vi "PAM v1.2.vi"() -> ()   [LabVIEW 2011]
uses:
  PAM_Control.ctl
  <vilib>/Utility/error.llb/DialogType.ctl
  <vilib>/Analysis/Matrix/Datatypes/RealMatrix.ctl
  <vilib>/DAQmx/read.llb/DAQmx Read (Analog 1D Wfm NChan NSamp).vi
  <vilib>/DAQmx/write.llb/DAQmx Write (Analog 1D DBL NChan 1Samp).vi
  PAM SubVIs/RH Probe Global Var.vi
  <vilib>/DAQmx/configure/timing.llb/DAQmx Timing (Sample Clock).vi
  <vilib>/Utility/file.llb/Write To Spreadsheet File (string).vi
  <vilib>/Analysis/Matrix/Numeric/Conversions/Matrix To Array - RM.vi
  <vilib>/DAQmx/miscellaneous.llb/DAQmx Fill In Error Info.vi
  Program Files (x86)/National Instruments/LabVIEW 2011/resource/objmgr/daqmx.rc
  <vilib>/Analysis/Matrix/NI_Matrix.lvlib
panel:
  out "O3 Data":sgl[](graph)
  out "SO2 Data":sgl[](graph)
  out "NO, NO2, NOx Data":dbl[][](graph)
  out "Bad Advantech Data Points":dbl
  out "Run In Progress?":bool
  out "Manual":bool
  in  "MFC Sequence File":path=path "C:/Users/PAM/Dropbox/Research - Dr. Williams/PAM/LabVIEW PAM/PAM Edited/defaultMFCSequence.txt"
  out "Auto":bool
  out "P Unit":string
  out "Pressure Transducer":dbl(knob) scale=1.9345053227622008e-18..193.3373735517042
  out "Error Out":errorcluster
  out "Elapsed Time (min)":dbl format="%#_2g"
  in  "Run Start Time":timestamp format="%<%X\n%x>T"
  out "NOx Units":string="LPM"
  in  "NOx Control (LPM)":dbl(slide) scale=0.0..0.04
  out "NOx Reading (LPM) 3":dbl(slide) scale=0.0..0.5
  out "VOC Units":string="LPM"
  in  "VOC Control (LPM)":dbl(slide) scale=0.0..0.5
  out "VOC Reading (LPM)":dbl(slide) scale=0.0..0.04
  out "O2 Units":string="LPM"
  in  "O2 Control (LPM)":dbl(slide) scale=0.0..1.0
  out "O2 Reading (LPM) 2":dbl(slide) scale=0.0..1.0 scale format="%#.2f"
  out "N2 Units":string="LPM"
  in  "N2 Control (LPM)":dbl(slide) scale=0.0..20.0
  out "N2 Reading (LPM)":dbl(slide) scale=0.0..20.0 scale format="%#.2f"
  out "AI (non TC) Units":string[](array[string])
  out "AI (non TC) Names":string[](array[string])
  out "RH Values":dbl[](array[numeric]) format="%#.2f"
  out "All Temp Units":i32[](array[ring]) items=["Deg C"=10143, "Deg F"=10144, "Kelvins"=10325, "Deg R"=10145, "From Custom Scale"=10065]
  out "All TC Labels":string[](array[string])
  out "TC Values Readings":dbl[](array[numeric]) format="%#_3g"
  out "Relative Humidity Data":waveform(dbl)[](graph) caption="Waveform Chart"
  in  "Stop Button":bool
  out "Temperature Data":dynamicdata(graph) caption="Waveform Chart"
  in  "Sampling Frequency (Hz)":dbl=5.0 caption="Delay Time (s)"
  in  "Trigger Type":T1(tab)
  in  "In Use? 11":bool=TRUE
  in  "In Use? 10":bool=TRUE
  in  "In Use? 9":bool=TRUE
  in  "In Use? 8":bool=TRUE
  in  "In Use? 7":bool=TRUE
  in  "In Use? 6":bool=TRUE
  in  "In Use? 5":bool=TRUE
  in  "Adv. TC 7":string="TC 7"
  in  "Adv. TC 6":string="TC 6"
  in  "Adv. TC 5":string="TC 5"
  in  "Adv. TC 4":string="TC 4"
  in  "Adv. TC 3":string="TC 3"
  in  "Adv. TC 2":string="TC 2"
  in  "Adv. TC 1":string="TC 1"
  in  "units":i32(ring)=10143 items=["Deg C"=10143, "Deg F"=10144, "Kelvins"=10325, "Deg R"=10145, "From Custom Scale"=10065]
  in  "In Use? 14":bool=TRUE
  in  "Physical Channel 14":tag="Dev1/ai7"
  in  "TC 14":string="PAM Downstream"
  in  "In Use? 13":bool=TRUE
  in  "Physical Channel 13":tag="Dev1/ai3"
  in  "TC 13":string="Humidifier"
  in  "In Use? 12":bool
  in  "Physical Channel 12":tag="Dev1/ai23"
  in  "TC 12":string="TC 12"
  in  "In Use? 15":bool
  in  "In Use? 14":bool
  in  "In Use? 13":bool
  in  "In Use? 12":bool
  in  "Physical Channel 4":tag="Dev1/ai21"
  in  "TC 4":string="TC 11"
  in  "Physical Channel 3":tag="Dev1/ai17"
  in  "TC 3":string="TC 10"
  in  "Physical Channel 2":tag="Dev1/ai20"
  in  "TC 2":string="TC 9"
  in  "Physical Channel":tag="Dev1/ai16"
  in  "TC 1":string="TC 8"
  in  "Thermocouple Type 1":T2=10073 items=["J"=10072, "K"=10073, "N"=10077, "R"=10082, "S"=10085, "T"=10086, "B"=10047, "E"=10055]
  in  "Min Value (deg C)":dbl
  in  "Max Value (deg C)":dbl=100.0
  in  "CJC Source":i32(ring)=10116 items=["Built-In"=10200, "Constant Value"=10116, "Channel"=10113]
  in  "CJC Value":dbl=25.0 format="%0.2f"
  in  "CJC Channel":refnum<k21>
  in  "In Use? 3":bool=TRUE
  in  "In Use? 4":bool=TRUE
  in  "RHT  2":tag="Dev1/ai5"
  in  "RHT Probe 2":string="RH 2"
  in  "RHT  1":tag="Dev1/ai4"
  in  "RHT Probe 1":string="RH 1"
  in  "In Use? 1":bool=TRUE
  in  "RHT  4":tag="Dev1/ai1"
  in  "RHT Probe 4":string="RHT T2"
  in  "RHT  3":tag="Dev1/ai0"
  in  "RHT Probe 3":string="RHT T1"
  in  "In Use? 2":bool=TRUE
  in  "Vaisala RH Scale":tag="RH Vaisala"
  in  "Vaisala T Scale":tag="RHT - Temp"
  in  "physical channels 4":tag="Dev1/ao3"
  out "Scale for VOC MFC 2":tag="NOx uMFC B"
  out "VOC MFC 2":string="VOC"
  in  "physical channels 3":tag="Dev1/ao2"
  out "Scale for NOx MFC 2":tag="NOx uMFC A"
  out "NOx MFC 2":string="NOx"
  in  "physical channels 2":tag="Dev1/ao1"
  out "Scale for O2 MFC 2":tag="O2 MFC B"
  out "O2 MFC 2":string="O2"
  in  "Scale for VOC MFC":tag="NOx uMFC B"
  in  "VOC MFC Channel":tag="Dev1/ai22"
  in  "VOC MFC":string="VOC"
  in  "Scale for NOx MFC":tag="NOx uMFC A"
  in  "NOx MFC Channel":tag="Dev1/ai18"
  in  "NOx MFC":string="NOx"
  in  "Scale for O2 MFC":tag="O2 MFC B"
  in  "O2 MFC Channel":tag="Dev1/ai6"
  in  "O2 MFC":string="O2"
  in  "Scale for N2 MFC":tag="N2 MFC A"
  in  "N2 MFC Channel":tag="Dev1/ai2"
  in  "N2 MFC":string="N2"
  out "Scale for N2 MFC 2":tag="N2 MFC A"
  out "N2 MFC 2":string="N2"
  in  "physical channels":tag="Dev1/ao0"
  in  "Units":enum16{"Torr", "Psia", "Bar", "kPa"}(ring)=enum."Psia"
  in  "In Use? 16":bool=TRUE
  in  "Pressure Transducer Channel":tag="Dev1/ai19"
  in  "Pressure Transducer Label":string="Pressure"
  in  "In Use? 18":bool=TRUE
  in  "Instrument 3":T3(ring)=enum."O3 (49i)"
  in  "In Use? 17":bool=TRUE
  in  "Instrument 2":T3(ring)=enum."SO2 (43i-TLE)"
  in  "In Use? 17":bool=TRUE
  in  "Instrument":T3(ring)
  in  "Frequency (Hz)":dbl=0.1
  in  "Log Thermo Data?":bool
  out "File Path for Gas Analyzer Data":string
  out "File Path for PAM Data":string
  in  "Header Information":string[][](array[string])
  in  "Delimeter":string="\t"
  in  "Log PAM Data?":bool
  in  "folder path for Data (dialog if empty) 2":path=path "C:/Users/PAM/Documents/PAM DATA/Data Auto"
  in  "Data Logging Interval (s)":dbl=2.0 caption="Delay Time (s)"
  # "Timing Settings"
  # "DAQ Setup & More"
  # "NOx MFC controls and indicators"
  # "VOC MFC controls and indicators"
  # "O2 MFC controls and indicators"
  # "N2 MFC controls and indicators"
  # "Analog Input (non TC) Readings"
  # "Thermocouple Readings"
  # "Currently Out Of Order :/"
  # "TC 1"
  # "Advantech ai0"
  # "TC 2"
  # "Advantech ai1"
  # "TC 3"
  # "Advantech ai2"
  # "TC 4"
  # "Advantech ai3"
  # "TC 5"
  # "Advantech ai4"
  # "TC 6"
  # "Advantech ai5"
  # "TC 7"
  # "Advantech ai6"
  # "TC 8"
  # "TC 9"
  # "TC 10"
  # "TC 11"
  # "TC 12"
  # "TC 13"
  # "TC 14"
  # "Vaisala RHT Probe (RH Settings)"
  # "Vaisala RHT Probe (Temp. Settings)"
  # "MFC Analog Input Setup"
  # "MFC Analog Ouput Setup"
  # "VOC MFC"
  # "NOx MFC"
  # "O2 MFC"
  # "VOC MFC"
  # "NOx MFC"
  # "O2 MFC"
  # "N2 MFC"
  # "N2 MFC"
  # "O3 [Model 49i]"
  # "SO2 [Model 43i-TLE]"
  # "NO, NO2, NOx [Model 42i-TL]"
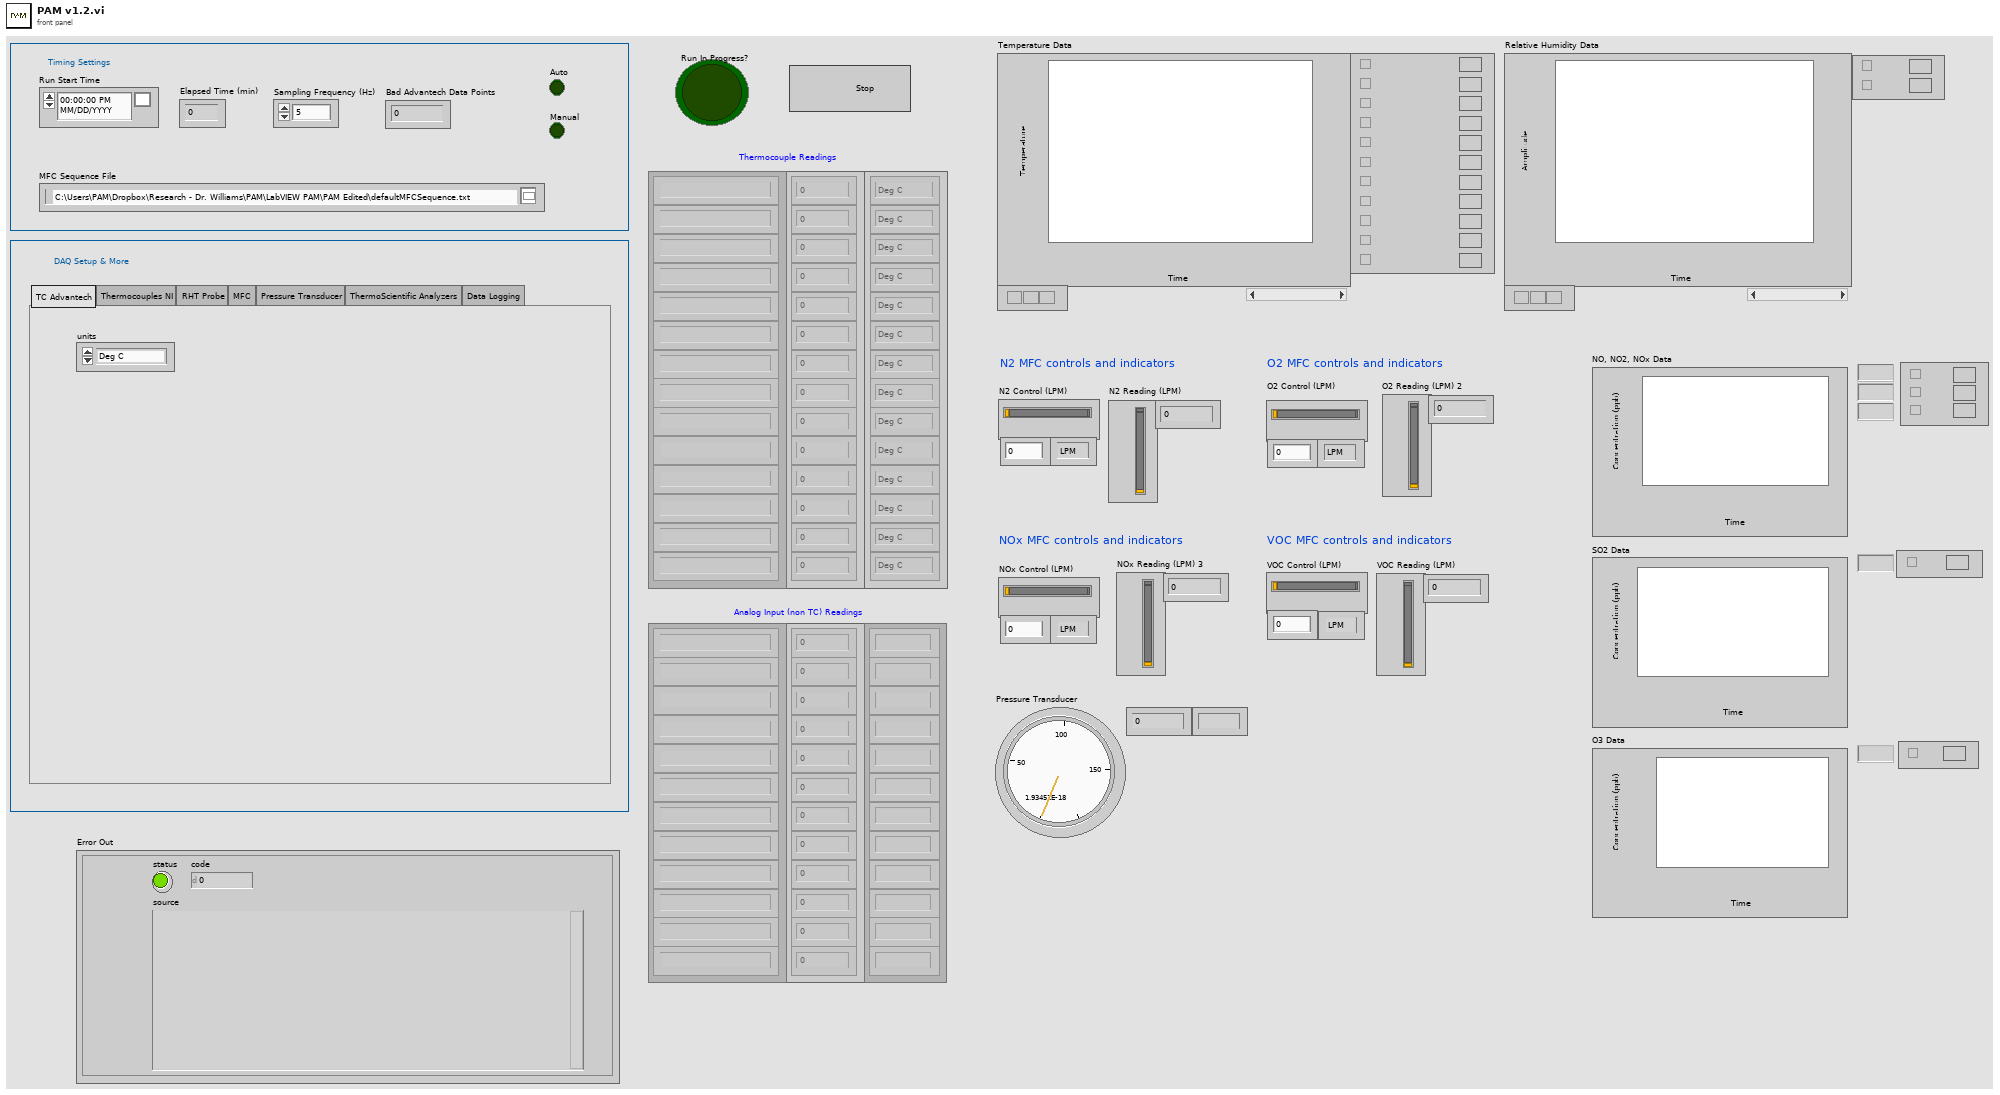
[diagram p1: front panel]
types:
  T1 = enum32{"TC Advantech", "Thermocouples NI", "RHT Probe", "MFC", "Pressure Transducer", "ThermoScientific Analyzers", "Data Logging"}
  T2 = typedef "PAM_Control.ctl" = i32
  T3 = enum16{"NOx (42i-TL)", "SO2 (43i-TLE)", "O3 (49i)"}
  T4 = cluster{"Label":string, "Boolean":bool, "Channel":tag, "Units":string, "Units Num":i32}[]
  T5 = cluster{"Label":string, "Channel":tag, "Scale":tag}[]
  T6 = cluster{"Label":string, "SP N2":dbl, "Time":dbl, "SP O2":dbl, "SP NOx":dbl, "SP VOC":dbl}[]
  T7 = typedef "NI_Matrix.lvlib/RealMatrix.ctl" = dbl[][]
  T8 = typedef "DialogType.ctl" = u16
  T9 = cluster{"Label":string, "Concentration":sgl, "Units":string}[]
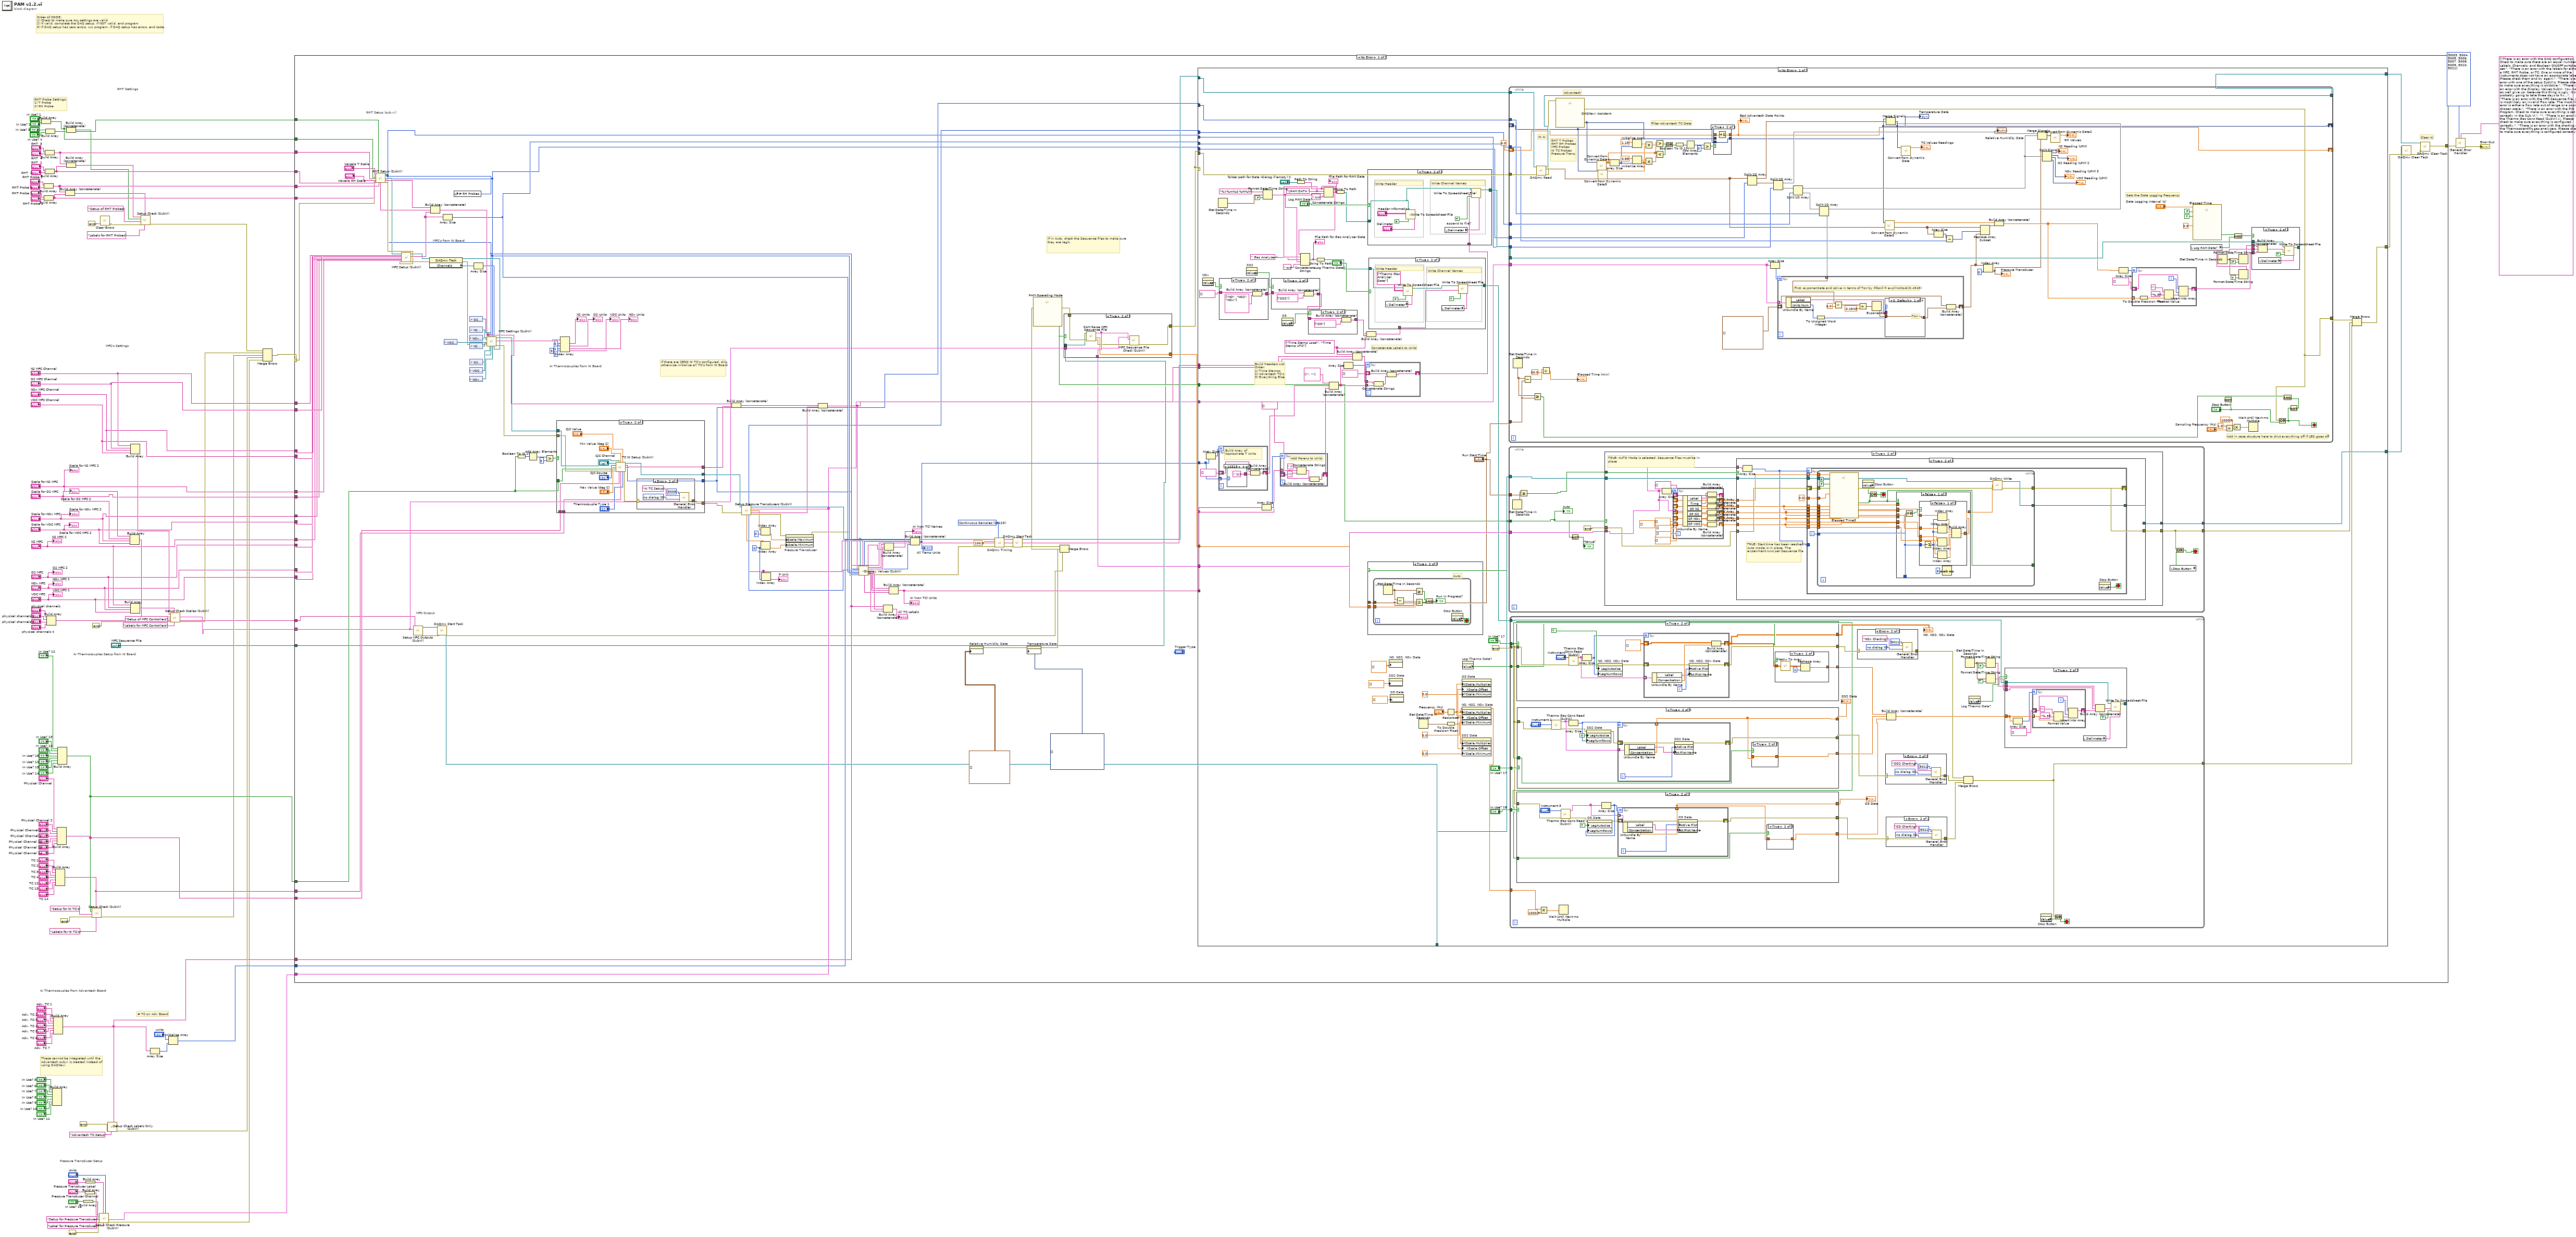
[diagram p0: block diagram]
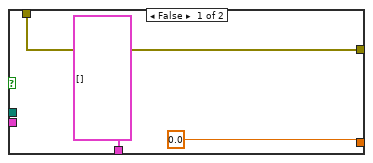
[diagram p2: hidden frame]
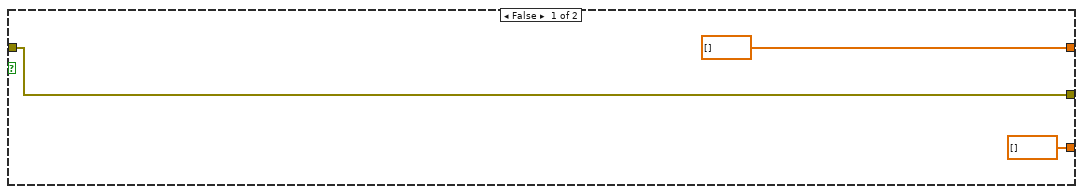
[diagram p11: hidden frame]
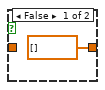
[diagram p12: hidden frame]
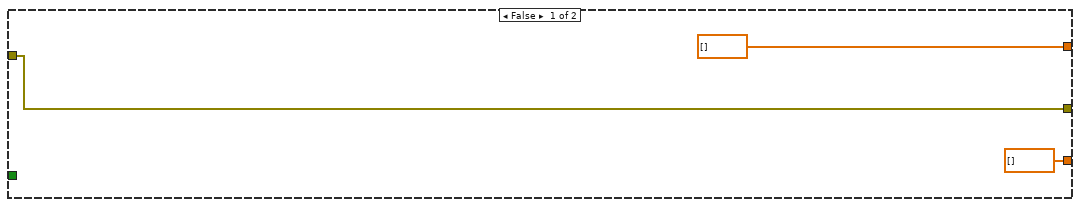
[diagram p13: hidden frame]
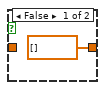
[diagram p14: hidden frame]
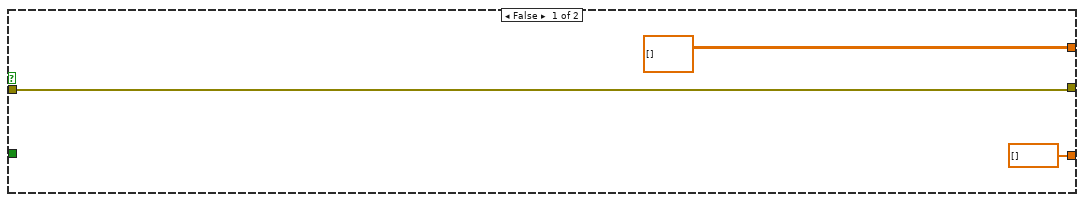
[diagram p15: hidden frame]
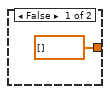
[diagram p16: hidden frame]
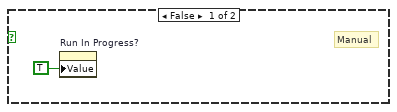
[diagram p17: hidden frame]
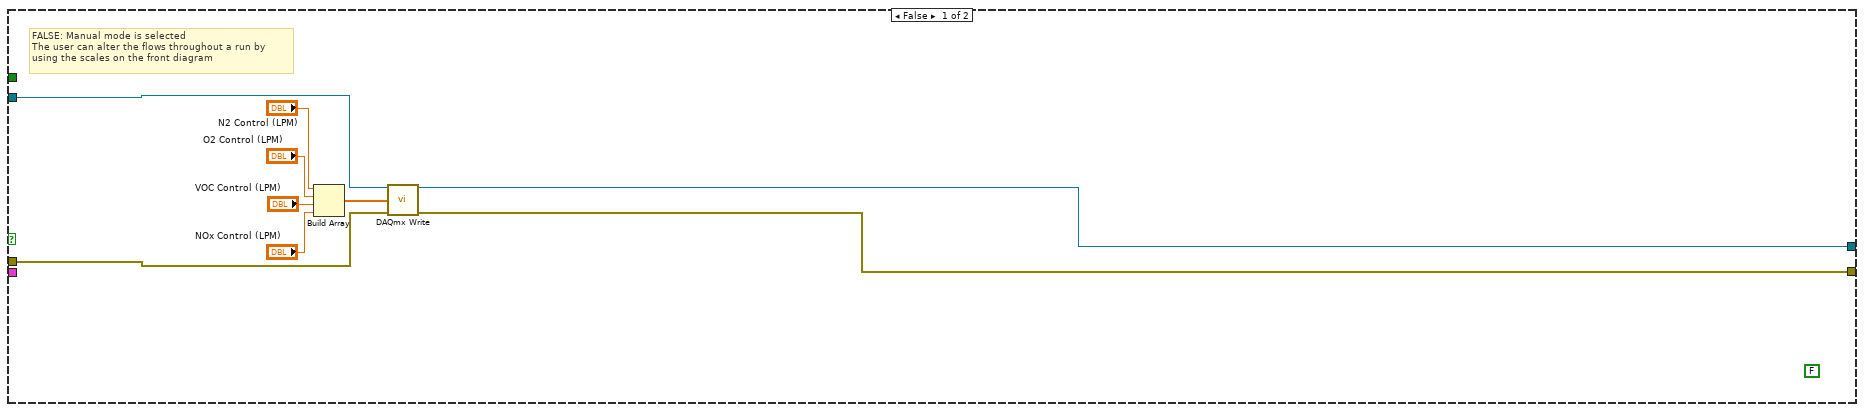
[diagram p18: hidden frame]
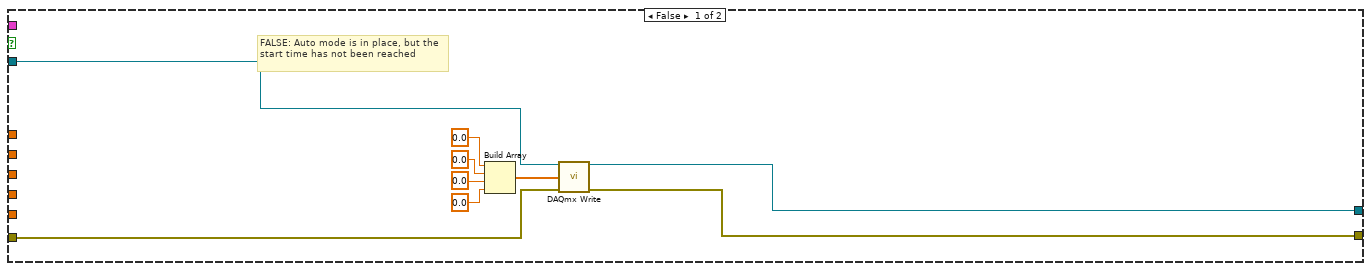
[diagram p19: hidden frame]
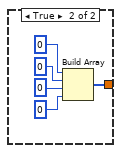
[diagram p20: hidden frame]
diagram:
  # "Pressure Transducer Setup"
  # "AI Thermocouples Setup from NI Board"
  # "MFC's Settings"
  # "Order of CODE:\n1) Check to make sure ALL settings are valid\n2) If valid, complete the DAQ setup. If NOT valid, end program\n3) If DAQ setup has zero errors, run program. If DAQ setup has errors, end code."
  # "RHT Probe Settings:\n1) T Probe\n2) RH Probe"
  # "These cannot be integrated until the Advantech subvi is created instead of using DAQNavi"
  # "RHT Settings"
  # "# TC on Adv Board"
  # "AI Thermocouples from Advantech Board"
  n1 = Build Array("In Use? 1", "In Use? 2") -> (w71:bool[])
  n2 = Build Array("RHT Probe 3", "RHT Probe 4") -> (w67:string[])
  n3 = Build Array("RHT Probe 1", "RHT Probe 2") -> (w66:string[])
  n4 = Build Array("RHT  3", "RHT  4") -> (w69:tag[])
  n5 = Build Array("RHT  1", "RHT  2") -> (w68:tag[])
  n6 = Build Array("In Use? 3", "In Use? 4") -> (w70:bool[])
  n7 = Build Array("physical channels", "physical channels 2", "physical channels 3", "physical channels 4") -> (w3:tag[])
  n8 = Build Array("In Use? 5", "In Use? 6", "In Use? 7", "In Use? 8", "In Use? 9", "In Use? 10", "In Use? 11") -> ()  [unwired: 1 out]
  n9 = Build Array("Adv. TC 1", "Adv. TC 2", "Adv. TC 3", "Adv. TC 4", "Adv. TC 5", "Adv. TC 6", "Adv. TC 7") -> (w38:string[])
  n10 = Build Array("TC 1", "TC 2", "TC 3", "TC 4", "TC 12", "TC 13", "TC 14") -> (w50:string[])
  n11 = Build Array("Physical Channel", "Physical Channel 2", "Physical Channel 3", "Physical Channel 4", "Physical Channel 12", "Physical Channel 13", "Physical Channel 14") -> (w51:tag[])
  n12 = Build Array("In Use? 12", "In Use? 13", "In Use? 14", "In Use? 15", "In Use? 12", "In Use? 13", "In Use? 14") -> (w52:bool[])
  n13 = Build Array (concatenate)(w67, w66) -> (w65:string[])
  n14 = Build Array (concatenate)(w69, w68) -> (w42:tag[])
  n15 = Build Array (concatenate)(w71, w70) -> (w41:bool[])
  n16 = Build Array("In Use? 16") -> (w32:bool[])
  n17 = Build Array("Pressure Transducer Channel") -> (w31:tag[])
  n18 = Build Array("Pressure Transducer Label") -> (w33:string[])
  n19 = call "Setup Check (SubVI).vi"("[error source] (\" \")"="Labels for NI TC's" ("[error source] (\" \")"), "Labels Array"=w50, "error in (no error)"=errorcluster {"status"=FALSE, "code"=0, "source"=""} ("error constant"), "[error source] (\" \") 2"="Setup for NI TC's" ("[error source] (\" \") 2"), "Boolean Array"=w52, "Channel Array"=w51) -> ("error out"=w46:errorcluster)  [unwired: 4 in, 1 out]
  n20 = call "Setup Check Pressure (SubVI).vi"("Units"="Units", "[error source] (\" \")"="Label for Pressure Transducer" ("[error source] (\" \")"), "Labels Array"=w33, "error in (no error)"=errorcluster {"status"=FALSE, "code"=0, "source"=""} ("error constant"), "[error source] (\" \") 2"="Setup for Pressure Transducer" ("[error source] (\" \") 2"), "Boolean Array"=w32, "Channel Array"=w31) -> ("error out"=w27:errorcluster, "Cluster Out"=w25:T4)  [unwired: 3 in]
  n21 = call <vilib>:"Clear Errors.vi"("error in (no error)"=errorcluster {"status"=FALSE, "code"=0, "source"=""} ("error constant")) -> ("error out"=w73:errorcluster)  [unwired: 6 in]
  n22 = call "Setup Check Labels Only (SubVI).vi"("error in (no error)"=errorcluster {"status"=FALSE, "code"=0, "source"=""} ("error constant"), "[error source] (\" \")"="Advantech TC Setup" ("[error source] (\" \")"), "Labels Array"=w38) -> ("error out"=w44:errorcluster)  [unwired: 6 in, 1 out]
  n23 = Build Array("Scale for N2 MFC", "Scale for O2 MFC", "Scale for NOx MFC", "Scale for VOC MFC") -> (w56:tag[])
  n24 = Build Array("N2 MFC Channel", "O2 MFC Channel", "NOx MFC Channel", "VOC MFC Channel") -> (w59:tag[])
  n25 = Build Array("N2 MFC", "O2 MFC", "NOx MFC", "VOC MFC") -> (w57:string[])
  n26 = call "Setup Check (SubVI).vi"("[error source] (\" \")"="Labels for RHT Probes" ("[error source] (\" \")"), "Labels Array"=w65, "error in (no error)"=w73, "[error source] (\" \") 2"="Setup of RHT Probes" ("[error source] (\" \")"), "Boolean Array"=w41, "Channel Array"=w42) -> ("error out"=w64:errorcluster)  [unwired: 4 in, 1 out]
  n27 = Array Size(array=w38) -> (size(s)=w102:i32)
  n28 = Initialize Array("units", w102) -> (w101:i32[])
  n29 = call "Setup Check Scales (SubVI).vi"("[error source] (\" \")"="Labels for MFC Controllers" ("[error source] (\" \")"), "Labels Array"=w57, "error in (no error)"=errorcluster {"status"=FALSE, "code"=0, "source"=""} ("error constant"), "[error source] (\" \") 2"="Setup of MFC Controllers" ("[error source] (\" \") 2"), "Scale Array"=w56, "Channel Array"=w59) -> ("error out"=w53:errorcluster, "Array of Clusters Out"=w2:T5)  [unwired: 4 in]
  n30 = Merge Errors(w64, w53, w46, w44, w27) -> (w39:errorcluster)
  n31 = case shown="No Error" w39 {
    selector: w39 -> [w145 w845]
    tunnel: w101 -> [w215 _]
    tunnel: [w198 w845] -> w89
    tunnel: w71 -> [w197 _]
    tunnel: w70 -> [w196 _]
    tunnel: w69 -> [w195 _]
    tunnel: w68 -> [w194 _]
    tunnel: w67 -> [w193 _]
    tunnel: w66 -> [w192 _]
    tunnel: "N2 MFC Channel" -> [w189 _]
    tunnel: "O2 MFC Channel" -> [w188 _]
    tunnel: "NOx MFC Channel" -> [w187 _]
    tunnel: "VOC MFC Channel" -> [w186 _]
    tunnel: "Scale for N2 MFC" -> [w185 _]
    tunnel: "Scale for O2 MFC" -> [w184 _]
    tunnel: "Scale for NOx MFC" -> [w183 _]
    tunnel: "Scale for VOC MFC" -> [w182 _]
    tunnel: "N2 MFC" -> [w181 _]
    tunnel: "O2 MFC" -> [w180 _]
    tunnel: "NOx MFC" -> [w179 _]
    tunnel: "VOC MFC" -> [w178 _]
    tunnel: w52 -> [w176 _]
    tunnel: w51 -> [w175 _]
    tunnel: w50 -> [w174 _]
    tunnel: w38 -> [w173 _]
    tunnel: w25 -> [w158 _]
    tunnel: w3 -> [w144 _]
    tunnel: w2 -> [w121 _]
    tunnel: "MFC Sequence File" -> [w124 _]
    frame No Error {
      w150 = 0 ("index")
      w204 = 10123 items=["Finite Samples"=10178, "Continuous Samples"=10123, "Hardware Timed Single Point"=12522] ("sample mode")
      # "If in Auto, check the Sequence files to make sure they are legit."
      # "MFC Output"
      # "RHT Setup (sub.vi)"
      # "If there are ZERO NI TC's configured, skip, otherwise initialize all TC's from NI Board"
      # "Clear AI"
      # "MFC's from NI Board"
      # "AI Thermocouples from NI Board"
      n32 = call "RHT Setup (SubVI).vi"("RH Used?"=w196, "Vaisala T Scale"="Vaisala T Scale", "Error In"=w145, "TC Used?"=w197, "RHT (T) Channels"=w195, "Vaisala RH Scale"="Vaisala RH Scale", "RH Names"=w192, "RH Channels"=w194, "RHT (T) Names"=w193) -> ("RH Labels"=w230:string[], "Refnum out"=w240:refnum<k21>, "# RH Probes"=w199:i32, "# RH (T) Probes"=w200:i32, "RH (T) Labels"=w233:string[], "error out"=w241:errorcluster)  [unwired: 13 in]
      n33 = call "MFC Setup (SubVI).vi"("Refnum in"=w240, "O2 MFC"=w180, "VOC MFC Channel"=w186, "Scale for VOC MFC"=w182, "NOx MFC"=w179, "error in (no error)"=w241, "NOx MFC Channel"=w187, "VOC MFC"=w178, "N2 MFC"=w181, "Scale for N2 MFC"=w185, "O2 MFC Channel"=w188, "Scale for O2 MFC"=w184, "N2 MFC Channel"=w189, "Scale for NOx MFC"=w183) -> ("Refnum out"=w238:refnum<k21>, "Array"=w213:string[], "error out"=w237:errorcluster)  [unwired: 3 in]
      n34 = call "Setup MFC Outputs (SubVI).vi"("Array of Clusters Out"=w121, "Array"=w144) -> ("error out"=w140:errorcluster, "Refnum out"=w137:refnum<k21>)  [unwired: 8 in]
      n35 = property class="DAQmx Task"(reference=w238, error in=w237) -> (reference out=w235:refnum<k21>, error out=w139:errorcluster, "Channels"=w234:refnum<k21>[])
      n36 = Build Array (concatenate)(w233, w230, w213) -> (w214:string[])
      n37 = call <vilib>:"DAQmx Start Task.vi"("task/channels in"=w137, "error in"=w140) -> ("task out"=w143:refnum<k21>, "error out"=w142:errorcluster)  [unwired: 12 in]
      n38 = Array Size(array=w213) -> (size(s)=w212:i32)
      n39 = control-ref of="VOC Reading (LPM)"() -> (w177:refnum<vi>)
      n40 = global write "RH Probe Global Var.vi" "# RH Probes"(w199) -> ()
      n41 = control-ref of="O2 Reading (LPM) 2"() -> (w221:refnum<vi>)
      n42 = control-ref of="N2 Reading (LPM)"() -> (w222:refnum<vi>)
      n43 = control-ref of="NOx Reading (LPM) 3"() -> (w220:refnum<vi>)
      n44 = control-ref of="N2 Control (LPM)"() -> (w219:refnum<vi>)
      n45 = control-ref of="O2 Control (LPM)"() -> (w218:refnum<vi>)
      n46 = control-ref of="VOC Control (LPM)"() -> (w217:refnum<vi>)
      n47 = control-ref of="NOx Control (LPM)"() -> (w216:refnum<vi>)
      n48 = Array Size(array=w234) -> (size(s)=w239:i32)
      n49 = call "MFC Settings (SubVI).vi"("Slide in"=w222, "Slide Refnum 3"=w220, "Channel Names"=w214, "Slide Refnum 4"=w177, "Slide Refnum 5"=w219, "error in (no error)"=w139, "Slide Refnum in"=w221, "Slide Refnum 6"=w218, "# RH Probes"=w199, "Slide Refnum 7"=w217, "# RH (T) Probes"=w200, "Slide Refnum 8"=w216, "# Channels"=w239, "task in"=w235) -> ("Refnum out"=w236:refnum<k21>, "MFC Units"=w136:string[], "error out"=w208:errorcluster)  [unwired: 3 in]
      n50 = Boolean To (0,1)(Boolean=w176) -> (0, 1=w209:i16[])
      n51 = Add Array Elements(numeric array=w209) -> (sum=w207:i16)
      n52 = Greater?(x=w207, y=i16 0) -> (0:w205:bool)
      n53 = case shown="True" w205 {
        tunnel: [w821 w823] -> w159
        tunnel: w236 -> [w822 w832]
        tunnel: [w822 w831] -> w167
        tunnel: w175 -> [_ w830]
        tunnel: w174 -> [_ w829]
        tunnel: [string[] [] ("Labels") w828] -> w211
        tunnel: [0 ("# TC (NI)") w827] -> w210
        tunnel: w176 -> [_ w826]
        tunnel: w208 -> [w821 w825]
        frame False {
        }
        frame True {
          n54 = call "TC NI Setup (SubVI).vi"("Refnum in"="CJC Channel", "Refnum out"=w832, "Min Value (deg C)"="Min Value (deg C)", "CJC Value"="CJC Value", "CJC Source"="CJC Source", "Max Value (deg C)"="Max Value (deg C)", "Boolean Array In"=w826, "error in (no error)"=w825, "Physical Channels"=w830, "Labels In"=w829, "Thermocouple Type 1"="Thermocouple Type 1") -> ("Refnum out"=w831:refnum<k21>, "# TC (NI)"=w827:i32, "Labels"=w828:string[], "error out"=w824:errorcluster)  [unwired: 1 in]
          n55 = case shown="Error" w824 {
            selector: w824 -> [w839 w843]
            tunnel: [w839 w844] -> w823
            frame No Error {
            }
            frame Error {
              w841 = T8 0 items=["no dialog", "OK message", "continue or stop message", "OK message + warnings", "continue/stop + warnings"] ("type of dialog (OK msg:1)")
              n56 = call <vilib>:"General Error Handler.vi"("[error code] (0)"=5005, "[error source] (\" \")"="AI TC Setup" ("[error source] (\" \")"), "type of dialog (OK msg:1)"=w841, "error in (no error)"=w843) -> ("error out"=w844:errorcluster)  [unwired: 7 in, 4 out]
            }
          }
        }
      }
      n57 = Index Array(array=w136, index #1=0 ("index"), index #2=1 ("index"), index #3=2 ("index"), index #4=3 ("index")) -> (element #1=→"N2 Units":string, element #2=→"O2 Units":string, element #3=→"NOx Units":string, element #4=→"VOC Units":string)
      n58 = Build Array (concatenate)(w214, w211) -> (w162:string[])
      n59 = call "Setup Pressure Transducers (SubVI).vi"("Refnum in"=w167, "Cluster Out"=w158, "Error In"=w159) -> ("Units"=w149:string[], "Refnum out"=w166:refnum<k21>, "Max Out"=w155:dbl[], "Array"=w163:string[], "Min Out"=w157:dbl[], "# Pressure Transducers"=w160:i32, "Error Out"=w153:errorcluster)  [unwired: 4 in, 2 out]
      n60 = Index Array(array=w155, index=0) -> (element=w152:dbl)
      n61 = Index Array(array=w157, index=w150) -> (element=w151:dbl)
      n62 = Index Array(array=w149, index=w150) -> (element=→"P Unit":string)
      n63 = property on="Pressure Transducer" class="Knob (strict)"(error in=w153, "Scale.Maximum"=w152, "Scale.Minimum"=w151) -> (error out=w154:errorcluster)  [unwired: 1 in, 1 out]
      n64 = Build Array (concatenate)(w162, w163) -> (w161:string[])
      n65 = call "Display Values (SubVI).vi"("Channels List"=w166, "All Names"=w161, "# PT"=w160, "# MFC"=w212, "# RH (T) Probes"=w200, "error In"=w154, "# TC (NI)"=w210, "# RH Probes"=w199, "PT Units In"=w149) -> ("NI TC Names"=w229:string[], "RH (T) Units"=w228:i32[], "PT Units Out"=w164:string[], "NI TC Units"=w172:i32[], "RH (T) Names"=w232:string[], "RH Names"=w226:string[], "MFC Names"=w224:string[], "PT Names"=w165:string[], "RH Units"=w225:string[], "MFC Units"=w223:string[], "error out"=w171:errorcluster)
      n66 = Build Array (concatenate)(w173, w232, w229) -> (→"All TC Labels":string[])
      n67 = Build Array (concatenate)(w226, w224, w165) -> (→"AI (non TC) Names":string[])
      n68 = Build Array (concatenate)(w225, w223, w164) -> (w146:string[])
      "AI (non TC) Units" <- w146
      n69 = Build Array (concatenate)(w215, w228, w172) -> (w147:i32[])
      "All Temp Units" <- w147
      n70 = property on="Relative Humidity Data" class="WFChart (strict)"("History Data"=waveform(dbl)[][] []) -> (error out=w243:errorcluster)  [unwired: 2 in, 1 out]
      n71 = call-poly <vilib>:"DAQmx Timing.vi"("task/channels in"=w166, "sample mode"=w204, "rate"=100.0, "error in"=w171) -> ("task out"=w202:refnum<k21>, "error out"=w170:errorcluster)  [unwired: 10 in]
      n72 = call <vilib>:"DAQmx Start Task.vi"("task/channels in"=w202, "error in"=w170) -> ("task out"=w201:refnum<k21>, "error out"=w169:errorcluster)  [unwired: 12 in]
      n73 = property on="Temperature Data" class="WFChart (strict)"(error in=w243, "History Data"=dynamicdata[] []) -> (error out=w242:errorcluster)  [unwired: 1 in, 1 out]
      n74 = Merge Errors(w169, w242, w142) -> (w138:errorcluster)
      n75 = call "PAM Operating Mode"("error in (no error)"=w138) -> ("Auto"=w127:bool, "error out"=w126:errorcluster)  [unwired: 17 in]
      n76 = case shown="True" w127 {
        tunnel: w126 -> [w248 w255]
        tunnel: [w248 w249] -> w125
        tunnel: w124 -> [_ w254]
        tunnel: [T6 [] ("Cluster Out") w252] -> w123
        tunnel: [0.0 ("Time (Last)") w253] -> w122
        tunnel: w121 -> [_ w250]
        frame False {
        }
        frame True {
          n77 = call "PAM Parse MFC Sequence File.vi"("error in"=w255, "Sequence File"=w254) -> ("error out"=w251:errorcluster, "Time (Last)"=w253:dbl, "Cluster Out"=w252:T6)  [unwired: 7 in]
          n78 = call "MFC Sequence File Check (SubVI).vi"("error in (no error)"=w251, "Sequence Cluster"=w252, "Cluster of MFCs"=w250) -> ("error in (no error) 2"=w249:errorcluster)  [unwired: 8 in]
        }
      }
      n79 = case shown="No Error" w125 {
        tunnel: w212 -> [w325 _]
        tunnel: w210 -> [w324 _]
        tunnel: w161 -> [w323 _]
        tunnel: w125 -> [w322 w818]
        tunnel: w201 -> [w321 w817]
        tunnel: w200 -> [w320 _]
        tunnel: w199 -> [w319 _]
        tunnel: w173 -> [w318 _]
        tunnel: [w317 w817] -> w168
        tunnel: [w297 w818] -> w120
        tunnel: w160 -> [w316 _]
        tunnel: w158 -> [w315 _]
        tunnel: w147 -> [w313 _]
        tunnel: w146 -> [w311 _]
        tunnel: w143 -> [w300 w816]
        tunnel: [w299 w816] -> w119
        tunnel: w127 -> [w294 _]
        tunnel: w123 -> [w295 _]
        tunnel: w122 -> [w292 _]
        frame No Error {
          w275 = "\\PAM DATA " ("string")
          w256 = string[] ["Time Stamp Local", "Time Stamp UTC"] ("array")
          # "Concatenate Labels to Units"
          # "Build Headers List \nOrder:\n1) Time Stamps\n2) Advantech TC's\n3) Everything Else"
          n80 = property on="NOx" class="Bool (strict)"() -> ("Value"=w267:bool)  [unwired: 2 in, 2 out]
          n81 = Array Size(array=w313) -> (size(s)=w314:i32)
          n82 = Get Date/Time In Seconds() -> (seconds since 1Jan1904=w331:timestamp)
          n83 = for {
            N: w314 -> [_]
            tunnel: w313 -> [w667] mode=indexing
            shift-right: [w666] -> w309
            shift-left: string[] [] -> [w664]
            # "Build Array of Appropriate T Units"
            n84 = case shown="10325" w667 {
              tunnel: [" (C)" " (F)" " (?)" " (K)" " (R)"] -> w665
              frame 10143 {
              }
              frame 10144 {
              }
              frame 10065, Default {
              }
              frame 10325 {
              }
              frame 10145 {
              }
            }
            n85 = Build Array (concatenate)(w664, w665) -> (w666:string[])
          }
          n86 = case shown="True" w267 {
            tunnel: [w342 w343] -> w264
            tunnel: string[] [] ("array") -> [w342 w344]
            frame False {
            }
            frame True {
              n87 = Build Array (concatenate)(w344, string[] ["NO", "NO2", "NOx"] ("array")) -> (w343:string[])
            }
          }
          n88 = property on="SO2" class="Bool (strict)"() -> ("Value"=w265:bool)  [unwired: 2 in, 2 out]
          n89 = Array Size(array=w311) -> (size(s)=w312:i32)
          n90 = Format Date/Time String(time format string (%c)="%Y%m%d %H%M", seconds (now)=w331, UTC format=FALSE) -> (date/time string=w271:string)
          n91 = case shown="True" w265 {
            tunnel: w264 -> [w338 w340]
            tunnel: [w338 w339] -> w263
            frame False {
            }
            frame True {
              n92 = Build Array (concatenate)(w340, string[] ["SO2"] ("array")) -> (w339:string[])
            }
          }
          n93 = for {
            N: w312 -> [_]
            tunnel: w311 -> [w663] mode=indexing
            shift-right: [w662] -> w308
            shift-left: string[] [] -> [w661]
            # "Add Parens to Units"
            n94 = Concatenate Strings(" (" ("string"), w663, ")" ("string")) -> (w660:string)
            n95 = Build Array (concatenate)(w661, w660) -> (w662:string[])
          }
          n96 = property on="O3" class="Bool (strict)"() -> ("Value"=w262:bool)  [unwired: 2 in, 2 out]
          n97 = Path To String(path="folder path for Data (dialog if empty) 2") -> (string=w274:string)
          n98 = Concatenate Strings(w274, w275, " Gas Analyzer " ("string"), w271, ".txt" ("string")) -> (w269:string)
          "File Path for Gas Analyzer Data" <- w269
          n99 = case shown="True" w262 {
            tunnel: w263 -> [w334 w336]
            tunnel: [w334 w335] -> w258
            frame False {
            }
            frame True {
              n100 = Build Array (concatenate)(w336, string[] ["O3"] ("array")) -> (w335:string[])
            }
          }
          n101 = String To Path(string=w269) -> (path=w268:path)
          n102 = Concatenate Strings(w274, w275, w271, ".txt" ("string")) -> (w276:string)
          "File Path for PAM Data" <- w276
          n103 = Build Array (concatenate)(string[] ["", ""], w309, w308) -> (w304:string[])
          n104 = String To Path(string=w276) -> (path=w327:path)
          n105 = Array Size(array=w304) -> (size(s)=w305:i32)
          n106 = Build Array (concatenate)(w256, w318, w323) -> (w303:string[])
          n107 = for {
            N: w305 -> [_]
            tunnel: w304 -> [w656] mode=indexing
            tunnel: w303 -> [w657] mode=indexing
            shift-right: [w655] -> w301
            shift-left: string[] [] -> [w653]
            n108 = Concatenate Strings(w657, w656) -> (w654:string)
            n109 = Build Array (concatenate)(w653, w654) -> (w655:string[])
          }
          n110 = Build Array (concatenate)(w256, w258) -> (w257:string[])
          n111 = case shown="True" "Log PAM Data?" {
            tunnel: w301 -> [_ w676]
            tunnel: w327 -> [w673 w675]
            tunnel: [w673 w674] -> w326
            frame False {
            }
            frame True {
              w679 = TRUE  # append to file?
              # "Write Channel Names"
              # "Write Header"
              n112 = call-poly <vilib>:"Write To Spreadsheet File.vi"("delimiter (\\t)"="Delimeter", "append to file? (new file:F)"=FALSE, "2D data"="Header Information", "file path (dialog if empty)"=w675) -> ()  [unwired: 4 in, 1 out]
              n113 = local read "Delimeter"() -> (w677:string)
              n114 = call-poly <vilib>:"Write To Spreadsheet File.vi"("delimiter (\\t)"=w677, "append to file? (new file:F)"=w679, "1D data"=w676, "file path (dialog if empty)"=w675) -> ("new file path (Not A Path if cancelled)"=w674:path)  [unwired: 3 in, 1 out]
            }
          }
          n115 = case shown="True" w294 {
            tunnel: "Run Start Time" -> [_ w498]
            tunnel: w292 -> [_ w497]
            frame False {
              # "Manual"
              n116 = property on="Run In Progress?" class="Bool (strict)"("Value"=TRUE ("Run In Progress?")) -> ()  [unwired: 2 in, 2 out]
            }
            frame True {
              # "Auto"
              n117 = while {
                tunnel: w498 -> [w504]
                tunnel: w497 -> [w503]
                stop <- w502 stop-if-true
                n118 = Get Date/Time In Seconds() -> (seconds since 1Jan1904=w505:timestamp)
                n119 = Subtract(x=w505, y=w504) -> (x-y=w500:dbl)
                n120 = Greater Or Equal?(x=w505, y=w504) -> (x >= y?=w506:bool)
                n121 = Less Or Equal?(x=w500, y=w503) -> (x <= y?=w501:bool)
                n122 = And(x=w506, y=w501) -> (x .and. y?=→"Run In Progress?":bool)
                n123 = property on="Stop Button" class="Bool (strict)"() -> ("Value"=w502:bool)  [unwired: 2 in, 2 out]
              }
            }
          }
          n124 = case shown="True" "Log Thermo Data?" {
            tunnel: w268 -> [w346 w352]
            tunnel: [w346 w348] -> w259
            tunnel: w257 -> [_ w347]
            frame False {
            }
            frame True {
              # "Write Header"
              # "Write Channel Names"
              n125 = local read "Delimeter"() -> (w355:string)
              n126 = call-poly <vilib>:"Write To Spreadsheet File.vi"("delimiter (\\t)"=w355, "append to file? (new file:F)"=FALSE, "2D data"=string[][] [["Thermo Gas Analyzer Data"]], "file path (dialog if empty)"=w352) -> ("new file path (Not A Path if cancelled)"=w351:path)  [unwired: 4 in]
              n127 = local read "Delimeter"() -> (w349:string)
              n128 = call-poly <vilib>:"Write To Spreadsheet File.vi"("delimiter (\\t)"=w349, "append to file? (new file:F)"=TRUE, "1D data"=w347, "file path (dialog if empty)"=w351) -> ("new file path (Not A Path if cancelled)"=w348:path)  [unwired: 3 in, 1 out]
            }
          }
          n129 = property on="SO2 Data" class="WFChart (strict)"("History Data"=sgl[] []) -> ()  [unwired: 2 in, 2 out]
          n130 = property on="NO, NO2, NOx Data" class="WFChart (strict)"("History Data"=dbl[][] []) -> ()  [unwired: 2 in, 2 out]
          n131 = property on="O3 Data" class="WFChart (strict)"("History Data"=sgl[] []) -> ()  [unwired: 2 in, 2 out]
          n132 = Get Date/Time In Seconds() -> (seconds since 1Jan1904=w282:timestamp)
          n133 = Reciprocal(x="Frequency (Hz)") -> (1/x=w280:dbl)
          n134 = To Double Precision Float(number=w282) -> (double precision float=w279:dbl)
          n135 = property on="O3 Data" class="WFChart (strict)"("XScale.Multiplier"=w280, "XScale.Offset"=w279, "YScale.Minimum"=0.0 ("Y Scale.Range:Minimum")) -> ()  [unwired: 2 in, 2 out]
          n136 = property on="NO, NO2, NOx Data" class="WFChart (strict)"("XScale.Multiplier"=w280, "XScale.Offset"=w279, "YScale.Minimum"=0.0 ("Y Scale.Range:Minimum")) -> ()  [unwired: 2 in, 2 out]
          n137 = property on="SO2 Data" class="WFChart (strict)"("XScale.Multiplier"=w280, "XScale.Offset"=w279, "YScale.Minimum"=0.0 ("Y Scale.Range:Minimum")) -> ()  [unwired: 2 in, 2 out]
          n138 = property on="Log Thermo Data?" class="Bool (strict)"() -> ("Value"=w260:bool)  [unwired: 2 in, 2 out]
          n139 = while {
            tunnel: w322 -> [w736]
            tunnel: w321 -> [w737]
            tunnel: [w765] -> w317
            tunnel: w324 -> [w724]
            tunnel: w325 -> [w762]
            tunnel: [w704] -> w298
            tunnel: w319 -> [w739]
            tunnel: w320 -> [w740]
            tunnel: "Run Start Time" -> [w755]
            tunnel: w326 -> [w752]
            tunnel: w316 -> [w713]
            tunnel: w315 -> [w720]
            shift-right: [w685] -> _
            shift-left: _ -> [w690]
            shift-right: [w682] -> _
            shift-left: 0.0 -> [w686]
            stop <- w768 stop-if-true
            # "Filter Advantech TC Data"
            # "Sets the Data Logging Frequency"
            # "Add in case structure here to shut everything off if LED goes off"
            # "RHT T Probes\nRHT RH Probes\nMFC Probes\nNI TC Probes\nPressure Trans."
            # "NI AI"
            # "Advantech"
            n140 = Get Date/Time In Seconds() -> (seconds since 1Jan1904=w754:timestamp)
            n141 = Subtract(x=w754, y=w755) -> (x-y=w707:dbl)
            n142 = Greater Or Equal?(x=w754, y=w755) -> (x >= y?=w710:bool)
            n143 = call-poly <vilib>:"DAQmx Read.vi"("task/channels in"=w737, "error in"=w736) -> ("task out"=w765:refnum<k21>, "data"=w683:waveform(dbl)[], "error out"=w745:errorcluster)  [unwired: 11 in]
            n144 = Divide(x=w707, y=60.0) -> (x/y=→"Elapsed Time (min)":dbl)
            n145 = call "DAQNavi Assistant"("error in(no error)"=w745) -> ("error out"=w704:errorcluster, "data out(DDT)"=w688:dynamicdata)  [unwired: 17 in]
            n146 = call "Convert from Dynamic Data4"("Dynamic Data Type"=w688) -> ("Array"=w684:dbl[])  [unwired: 3 in]
            n147 = call "Convert from Dynamic Data5"("Dynamic Data Type"=w690) -> ("Array"=w689:dbl[])  [unwired: 3 in]
            n148 = Array Size(array=w684) -> (size(s)=w696:i32)
            n149 = Initialize Array(1.15 ("element"), w696) -> (w703:dbl[])
            n150 = Initialize Array(0.85 ("element"), w696) -> (w702:dbl[])
            n151 = Multiply(x=w703, y=w689) -> (x*y=w694:dbl[])
            n152 = Multiply(x=w702, y=w689) -> (x*y=w693:dbl[])
            n153 = Greater?(x=w684, y=w694) -> (0:w701:bool[])
            n154 = Less?(x=w684, y=w693) -> (x < y?=w687:bool[])
            n155 = Or(x=w701, y=w687) -> (x .or. y?=w692:bool[])
            n156 = Boolean To (0,1)(Boolean=w692) -> (0, 1=w691:i16[])
            n157 = Add Array Elements(numeric array=w691) -> (sum=w700:i16)
            n158 = Greater?(x=w700, y=i16 0) -> (0:w695:bool)
            n159 = case shown="True" w695 {
              tunnel: w688 -> [w772 _]
              tunnel: [w772 w775] -> w685
              tunnel: w690 -> [_ w775]
              tunnel: [w771 w774] -> w682
              tunnel: w686 -> [w771 w773]
              frame False {
              }
              frame True {
                n160 = Increment(x=w773) -> (x+1=w774:dbl)
              }
            }
            "Bad Advantech Data Points" <- w682
            n161 = Split 1D Array(array=w683, index=w740) -> (first subarray=w758:waveform(dbl)[], second subarray=w767:waveform(dbl)[])
            n162 = Array Size(array=w720) -> (size(s)=w717:i32)
            n163 = Split 1D Array(array=w767, index=w739) -> (first subarray=w757:waveform(dbl)[], second subarray=w766:waveform(dbl)[])
            "Relative Humidity Data" <- w757
            n164 = Split 1D Array(array=w766, index=w762) -> (first subarray=w756:waveform(dbl)[], second subarray=w723:waveform(dbl)[])
            n165 = Split 1D Array(array=w723, index=w724) -> (first subarray=w722:waveform(dbl)[], second subarray=w721:waveform(dbl)[])
            n166 = for {
              N: w717 -> [_]
              tunnel: w721 -> [w785] mode=indexing
              tunnel: w720 -> [w788] mode=indexing
              shift-right: [w779] -> w715
              shift-left: waveform(dbl)[] [] -> [w778]
              # "First, exponentiate and solve in terms of Torr by P[torr] = exp((Volts-6)/0.4343)"
              n167 = Unbundle By Name(w788) -> ("Label"=w776:string, "Units Num"=w787:i32)
              n168 = To Unsigned Word Integer(number=w787) -> (unsigned 16bit integer=w786:u16)
              n169 = Subtract(x=w785, y=6.0) -> (x-y=w783:waveform(dbl))
              n170 = Divide(x=w783, y=0.4343) -> (x/y=w781:waveform(dbl))
              n171 = Exponential(1:w781) -> (0:w780:waveform(dbl))
              n172 = case shown="0, Default" w786 {
                tunnel: w776 -> [_ _ _ _]
                tunnel: w780 -> [w789 w792 w795 w798]
                tunnel: [w789 w791 w794 w797] -> w777
                frame 0, Default {
                  # "Torr"
                }
                frame 1 {
                  # "Psia"
                  n173 = Multiply(x=w792, y=0.0193396) -> (x*y=w791:waveform(dbl))
                }
                frame 2 {
                  # "Bar"
                  n174 = Multiply(x=w795, y=0.001333) -> (x*y=w794:waveform(dbl))
                }
                frame 3 {
                  # "kPa"
                  n175 = Multiply(x=w798, y=0.1333) -> (x*y=w797:waveform(dbl))
                }
              }
              n176 = Build Array (concatenate)(w778, w777) -> (w779:waveform(dbl)[])
            }
            n177 = call "Convert from Dynamic Data3"("Dynamic Data Type"=w685) -> ("Array"=w742:dbl[])  [unwired: 3 in]
            n178 = Merge Signals(w685, w758, w722) -> (w746:dynamicdata)
            "Temperature Data" <- w746
            n179 = call "Convert from Dynamic Data"("Dynamic Data Type"=w746) -> ("Array"=→"TC Values Readings":dbl[])  [unwired: 3 in]
            n180 = Array Size(array=w683) -> (size(s)=w714:i32)
            n181 = Subtract(x=w714, y=w713) -> (x-y=w711:i32)
            n182 = Replace Array Subset(array=w683, new element=w715, index=w711) -> (w712:waveform(dbl)[])
            n183 = Index Array(array=w715, index=0) -> (element=w716:waveform(dbl))
            "Pressure Transducer" <- w716
            n184 = Build Array (concatenate)(w742, w712) -> (w741:dbl[])
            n185 = Merge Signals(w757, w756, w716) -> (w763:dynamicdata)
            n186 = Split Signals(w756) -> (→"N2 Reading (LPM)":dynamicdata, →"O2 Reading (LPM) 2":dynamicdata, →"NOx Reading (LPM) 3":dynamicdata, →"VOC Reading (LPM)":dynamicdata)  [unwired: 4 in]
            n187 = call "Convert from Dynamic Data2"("Dynamic Data Type"=w763) -> ("Array"=→"RH Values":dbl[])  [unwired: 3 in]
            n188 = Array Size(array=w741) -> (size(s)=w744:i32)
            n189 = for {
              N: w744 -> [_]
              shift-right: [w805] -> w735
              shift-left: string[] [] -> [w803]
              tunnel: w741 -> [w799] mode=indexing
              i -> [w806]
              n190 = To Double Precision Float(number=w799) -> (double precision float=w802:dbl)
              n191 = Format Value(string ("")="", format string="%.3f", value (0)=w802) -> (output string=w804:string)
              n192 = Insert Into Array(array=w803, index=w806, new element=w804) -> (w805:string[])
            }
            n193 = local read "Log PAM Data?"() -> (w734:bool)
            n194 = call "Elapsed Time"("Time Target (s)"="Data Logging Interval (s)", "Reset"=FALSE, "Auto Reset"=TRUE, "Set Start Time (s)"=0.0) -> ("Time has Elapsed"=w733:bool)  [unwired: 8 in, 7 out]
            n195 = Get Date/Time In Seconds() -> (seconds since 1Jan1904=w750:timestamp)
            n196 = Not(x="Stop Button") -> ()  [unwired: 1 out]
            n197 = Divide(x=1.0, y="Sampling Frequency (Hz)") -> (x/y=w727:dbl)
            n198 = Multiply(x=1000.0, y=w727) -> (x*y=w725:dbl)
            n199 = And(x=w733, y=w734) -> (x .and. y?=w731:bool)
            n200 = Format Date/Time String(seconds (now)=w750, UTC format=FALSE ("to UTC (F)")) -> (date/time string=w747:string)  [unwired: 1 in]
            n201 = Format Date/Time String(seconds (now)=w750, UTC format=TRUE ("to UTC (F)")) -> (date/time string=w748:string)  [unwired: 1 in]
            n202 = Wait Until Next ms Multiple(millisecond multiple=w725) -> ()  [unwired: 1 out]
            n203 = case shown="True" w731 {
              tunnel: w752 -> [w807 w815]
              tunnel: [w807 w814] -> _
              tunnel: w748 -> [_ w810]
              tunnel: w747 -> [_ w809]
              tunnel: w735 -> [_ w808]
              frame False {
              }
              frame True {
                n204 = Build Array (concatenate)(w809, w810, w808) -> (w811:string[])
                n205 = local read "Delimeter"() -> (w813:string)
                n206 = call-poly <vilib>:"Write To Spreadsheet File.vi"("delimiter (\\t)"=w813, "append to file? (new file:F)"=TRUE, "1D data"=w811, "file path (dialog if empty)"=w815) -> ("new file path (Not A Path if cancelled)"=w814:path)  [unwired: 3 in, 1 out]
              }
            }
            n207 = Or(x=w704, y="Stop Button") -> (x .or. y?=w768:bool)
            n208 = Not(x=w768) -> (.not. x?=w753:bool)
            n209 = And(x=w710, y=w753) -> ()  [unwired: 1 out]
          }
          n210 = while {
            tunnel: w300 -> [w518]
            tunnel: "Run Start Time" -> [w509]
            tunnel: [w516] -> w299
            tunnel: [w515] -> w296
            tunnel: w294 -> [w511]
            tunnel: w295 -> [w512]
            stop <- w508 stop-if-true
            n211 = Get Date/Time In Seconds() -> (seconds since 1Jan1904=w510:timestamp)
            n212 = Greater Or Equal?(x=w510, y=w509) -> (x >= y?=w507:bool)
            n213 = Not(x=w511) -> (.not. x?=→"Manual":bool)
            n214 = case shown="True" w511 {
              tunnel: w518 -> [w525 w545]
              tunnel: [w527 w544] -> w516
              tunnel: [w519 w543] -> w515
              tunnel: errorcluster {"status"=FALSE, "code"=0, "source"=""} ("error in") -> [w526 w529]
              tunnel: w507 -> [_ w528]
              tunnel: w512 -> [_ w530]
              frame False {
                (unwired) FALSE ("Boolean")
                # "FALSE: Manual mode is selected\nThe user can alter the flows throughout a run by using the scales on the front diagram"
                n215 = Build Array("N2 Control (LPM)", "O2 Control (LPM)", "VOC Control (LPM)", "NOx Control (LPM)") -> (w524:dbl[])
                n216 = call-poly <vilib>:"DAQmx Write.vi"("task/channels in"=w525, "data"=w524, "error in"=w526) -> ("task out"=w527:refnum<k21>, "error out"=w519:errorcluster)  [unwired: 10 in, 1 out]
              }
              frame True {
                # "TRUE: AUTO Mode is selected. Sequence files must be in place"
                n217 = Array Size(array=w530) -> (size(s)=w542:i32)
                n218 = for {
                  N: w542 -> [_]
                  tunnel: w530 -> [w564] mode=indexing
                  shift-right: [w562] -> _
                  shift-left: string[] [] -> [w561]
                  shift-right: [w559] -> w535
                  shift-left: dbl[] [] -> [w558]
                  shift-right: [w556] -> w534
                  shift-left: dbl[] [] -> [w555]
                  shift-right: [w553] -> w533
                  shift-left: dbl[] [] -> [w552]
                  shift-right: [w550] -> w532
                  shift-left: dbl[] [] -> [w549]
                  shift-right: [w547] -> w531
                  shift-left: dbl[] [] -> [w546]
                  n219 = Unbundle By Name(w564) -> ("Label"=w563:string, "Time"=w560:dbl, "SP N2"=w557:dbl, "SP O2"=w554:dbl, "SP NOx"=w551:dbl, "SP VOC"=w548:dbl)
                  n220 = Build Array (concatenate)(w561, w563) -> (w562:string[])
                  n221 = Build Array (concatenate)(w558, w560) -> (w559:dbl[])
                  n222 = Build Array (concatenate)(w555, w557) -> (w556:dbl[])
                  n223 = Build Array (concatenate)(w552, w554) -> (w553:dbl[])
                  n224 = Build Array (concatenate)(w549, w551) -> (w550:dbl[])
                  n225 = Build Array (concatenate)(w546, w548) -> (w547:dbl[])
                }
                n226 = case shown="True" w528 {
                  tunnel: w545 -> [w568 w582]
                  tunnel: [w567 w577] -> w544
                  tunnel: [w566 w576] -> w543
                  tunnel: w529 -> [w565 w584]
                  tunnel: w530 -> [_ w585]
                  tunnel: w535 -> [_ w583]
                  tunnel: w534 -> [_ w581]
                  tunnel: w533 -> [_ w580]
                  tunnel: w532 -> [_ w579]
                  tunnel: w531 -> [_ w578]
                  frame False {
                    # "FALSE: Auto mode is in place, but the start time has not been reached"
                    n227 = Build Array(0.0 ("element"), 0.0 ("element"), 0.0 ("element"), 0.0 ("element")) -> (w569:dbl[])
                    n228 = call-poly <vilib>:"DAQmx Write.vi"("task/channels in"=w568, "data"=w569, "error in"=w565) -> ("task out"=w567:refnum<k21>, "error out"=w566:errorcluster)  [unwired: 10 in, 1 out]
                  }
                  frame True {
                    # "TRUE: Start time has been reached. Auto mode is in place. The experiment runs per Sequence file"
                    n229 = Array Size(array=w585) -> (size(s)=w574:i32)
                    n230 = for {
                      N: w574 -> [_]
                      tunnel: 0.0 ("Set Start Time (s)") -> [w601]
                      shift-right: [w592] -> w576
                      shift-left: w584 -> [w600]
                      tunnel: w583 -> [w599] mode=indexing
                      tunnel: w578 -> [w595] mode=indexing
                      tunnel: w579 -> [w596] mode=indexing
                      tunnel: w580 -> [w597] mode=indexing
                      tunnel: w581 -> [w598] mode=indexing
                      tunnel: w582 -> [w594]
                      tunnel: [w593] -> w577
                      tunnel: w581 -> [w591]
                      tunnel: w580 -> [w590]
                      tunnel: w579 -> [w589]
                      tunnel: w578 -> [w588]
                      tunnel: w574 -> [_]
                      i -> [w587]
                      stop <- w586 stop-if-true
                      n231 = while {
                        tunnel: w601 -> [w621]
                        tunnel: w600 -> [w620]
                        tunnel: w599 -> [w619]
                        tunnel: w598 -> [w618]
                        tunnel: w597 -> [w617]
                        tunnel: w596 -> [w616]
                        tunnel: w595 -> [w615]
                        tunnel: w594 -> [w614]
                        tunnel: [w613] -> w593
                        tunnel: [w612] -> w592
                        tunnel: w587 -> [w609]
                        tunnel: w591 -> [w608]
                        tunnel: w590 -> [w607]
                        tunnel: w589 -> [w606]
                        tunnel: w588 -> [w605]
                        tunnel: [w603] -> _
                        stop <- w602 stop-if-true
                        n232 = call "Elapsed Time3"("Time Target (s)"=w619, "Reset"=FALSE, "Auto Reset"=FALSE, "error in (no error)"=w620, "Set Start Time (s)"=w621) -> ("Time has Elapsed"=w603:bool, "error out"=w611:errorcluster)  [unwired: 7 in, 6 out]
                        n233 = property on="Stop Button" class="Bool (strict)"() -> ("Value"=w604:bool)  [unwired: 2 in, 2 out]
                        n234 = Or(x=w604, y=w603) -> (x .or. y?=w602:bool)
                        n235 = case shown="False" w603 {
                          tunnel: w618 -> [_ w652]
                          tunnel: w617 -> [_ w651]
                          tunnel: w616 -> [_ w650]
                          tunnel: w615 -> [_ w649]
                          tunnel: [w630 w648] -> w610
                          tunnel: w609 -> [w625 _]
                          tunnel: w608 -> [w629 _]
                          tunnel: w607 -> [w628 _]
                          tunnel: w606 -> [w627 _]
                          tunnel: w605 -> [w626 _]
                          frame False {
                            n236 = Equal To 0?(x=w625) -> (x = 0?=w631:bool)
                            n237 = case shown="False" w631 {
                              tunnel: [w637 w645] -> w630
                              tunnel: w629 -> [w642 _]
                              tunnel: w628 -> [w636 _]
                              tunnel: w627 -> [w635 _]
                              tunnel: w626 -> [w634 _]
                              tunnel: w625 -> [w633 _]
                              frame False {
                                n238 = Decrement(x=w633) -> (x-1=w632:i32)
                                n239 = Index Array(array=w642, index=w632) -> (element=w641:dbl)
                                n240 = Index Array(array=w636, index=w632) -> (element=w640:dbl)
                                n241 = Index Array(array=w635, index=w632) -> (element=w639:dbl)
                                n242 = Index Array(array=w634, index=w632) -> (element=w638:dbl)
                                n243 = Build Array(w641, w640, w639, w638) -> (w637:dbl[])
                              }
                              frame True {
                                n244 = Build Array(0, 0, 0 ("element"), 0 ("element")) -> (w645:i32[])
                              }
                            }
                            n245 = Wait (ms)(milliseconds to wait=u32 5) -> ()  [unwired: 1 out]
                          }
                          frame True {
                            n246 = Build Array(w652, w651, w650, w649) -> (w648:dbl[])
                          }
                        }
                        n247 = call-poly <vilib>:"DAQmx Write.vi"("task/channels in"=w614, "data"=w610, "error in"=w611) -> ("task out"=w613:refnum<k21>, "error out"=w612:errorcluster)  [unwired: 10 in, 1 out]
                      }
                      n248 = property on="Stop Button" class="Bool (strict)"() -> ("Value"=w586:bool)  [unwired: 2 in, 2 out]
                    }
                  }
                }
              }
            }
            n249 = local read "Stop Button"() -> (w514:bool)
            n250 = Or(x=w515, y=w514) -> (x .or. y?=w508:bool)
            "Auto" <- w511
          }
          n251 = while {
            tunnel: errorcluster {"status"=FALSE, "code"=0, "source"=""} ("Error In") -> [w382]
            tunnel: [w381] -> w261
            tunnel: "In Use? 17" -> [w365]
            tunnel: "In Use? 18" -> [w384]
            tunnel: "In Use? 17" -> [w383]
            tunnel: w280 -> [w372]
            tunnel: w260 -> [w370]
            tunnel: w259 -> [w358]
            stop <- w386 stop-if-true
            n252 = case shown="True" w365 {
              tunnel: [w470 w478] -> w380
              tunnel: w382 -> [w470 w481]
              tunnel: [T7 [] ("Real Matrix") w472] -> w371
              tunnel: w370 -> [_ w473]
              tunnel: [dbl[] [] ("Real 2D Array") w471] -> w368
              frame False {
              }
              frame True {
                n253 = call "Thermo Gas Conc Read (SubVI).vi"("Error In"=w481, "Instrument"="Instrument") -> ("error out"=w475:errorcluster, "Data Out"=w480:T9)  [unwired: 8 in]
                n254 = Array Size(array=w480) -> (size(s)=w476:i32)
                n255 = property on="NO, NO2, NOx Data" class="WFChart (strict)"(error in=w475, "LegAutosize"=TRUE ("Legend:Autosize"), "LegNumRows"=w476) -> (error out=w474:errorcluster)  [unwired: 1 in, 1 out]
                n256 = for {
                  N: w476 -> [_]
                  tunnel: w480 -> [w495] mode=indexing
                  shift-right: [w493] -> w472
                  shift-left: T7 [] ("Real Matrix") -> [w492]
                  shift-right: [w489] -> w478
                  shift-left: w474 -> [w488]
                  i -> [w491]
                  n257 = Unbundle By Name(w495) -> ("Label"=w490:string, "Concentration"=w494:sgl)
                  n258 = property on="NO, NO2, NOx Data" class="WFChart (strict)"(error in=w488, "Active Plot"=w491, "Plot.Plot Name"=w490) -> (error out=w489:errorcluster)  [unwired: 1 in, 1 out]
                  n259 = Build Array (concatenate)(w492, w494) -> (w493:T7)
                }
                n260 = case shown="True" w473 {
                  tunnel: w472 -> [_ w487]
                  tunnel: [dbl[] [] ("Real 2D Array") w484] -> w471
                  frame False {
                  }
                  frame True {
                    n261 = call-poly <vilib>:"Matrix To Array.vi"("Real Matrix"=w487) -> ("Real 2D Array"=w486:dbl[][])
                    n262 = Reshape Array(w486, 1 ("dimension size")) -> (w484:dbl[])
                  }
                }
              }
            }
            "NO, NO2, NOx Data" <- w371
            n263 = case shown="True" w384 {
              tunnel: w382 -> [w426 w436]
              tunnel: [w426 w430] -> w376
              tunnel: [sgl[] [] w428] -> w366
              tunnel: w365 -> [_ w429]
              tunnel: [sgl[] [] w427] -> w364
              frame False {
              }
              frame True {
                n264 = call "Thermo Gas Conc Read (SubVI).vi"("Error In"=w436, "Instrument"="Instrument 3") -> ("error out"=w435:errorcluster, "Data Out"=w434:T9)  [unwired: 8 in]
                n265 = Array Size(array=w434) -> (size(s)=w433:i32)
                n266 = property on="O3 Data" class="WFChart (strict)"(error in=w435, "LegAutosize"=TRUE ("Legend:Autosize"), "LegNumRows"=w433) -> (error out=w431:errorcluster)  [unwired: 1 in, 1 out]
                n267 = for {
                  N: w433 -> [_]
                  tunnel: w434 -> [w445] mode=indexing
                  tunnel: [w443] -> w428 mode=indexing
                  shift-right: [w441] -> w430
                  shift-left: w431 -> [w440]
                  i -> [w442]
                  n268 = Unbundle By Name(w445) -> ("Label"=w444:string, "Concentration"=w443:sgl)
                  n269 = property on="O3 Data" class="WFChart (strict)"(error in=w440, "Active Plot"=w442, "Plot.Plot Name"=w444) -> (error out=w441:errorcluster)  [unwired: 1 in, 1 out]
                }
                n270 = case shown="True" w429 {
                  tunnel: w428 -> [_ w439]
                  tunnel: [sgl[] [] w439] -> w427
                  frame False {
                  }
                  frame True {
                  }
                }
              }
            }
            "O3 Data" <- w366
            n271 = case shown="True" w383 {
              tunnel: w382 -> [w448 w458]
              tunnel: [w448 w456] -> w377
              tunnel: [sgl[] [] w450] -> w378
              tunnel: w365 -> [_ w451]
              tunnel: [sgl[] [] w449] -> w367
              frame False {
              }
              frame True {
                n272 = call "Thermo Gas Conc Read (SubVI).vi"("Error In"=w458, "Instrument"="Instrument 2") -> ("error out"=w453:errorcluster, "Data Out"=w457:T9)  [unwired: 8 in]
                n273 = Array Size(array=w457) -> (size(s)=w454:i32)
                n274 = property on="SO2 Data" class="WFChart (strict)"(error in=w453, "LegAutosize"=TRUE ("Legend:Autosize"), "LegNumRows"=w454) -> (error out=w452:errorcluster)  [unwired: 1 in, 1 out]
                n275 = for {
                  N: w454 -> [_]
                  tunnel: w457 -> [w467] mode=indexing
                  shift-right: [w464] -> w456
                  shift-left: w452 -> [w463]
                  tunnel: [w462] -> w450 mode=indexing
                  i -> [w466]
                  n276 = Unbundle By Name(w467) -> ("Label"=w465:string, "Concentration"=w462:sgl)
                  n277 = property on="SO2 Data" class="WFChart (strict)"(error in=w463, "Active Plot"=w466, "Plot.Plot Name"=w465) -> (error out=w464:errorcluster)  [unwired: 1 in, 1 out]
                }
                n278 = case shown="True" w451 {
                  tunnel: w450 -> [_ w461]
                  tunnel: [sgl[] [] w461] -> w449
                  frame False {
                  }
                  frame True {
                  }
                }
              }
            }
            "SO2 Data" <- w378
            n279 = Multiply(x=w372, y=1000.0) -> (x*y=w373:dbl)
            n280 = Wait Until Next ms Multiple(millisecond multiple=w373) -> ()  [unwired: 1 out]
            n281 = case shown="Error" w380 {
              selector: w380 -> [w418 w423]
              tunnel: [w418 w422] -> w379
              frame No Error {
              }
              frame Error {
                w419 = T8 0 items=["no dialog", "OK message", "continue or stop message", "OK message + warnings", "continue/stop + warnings"] ("type of dialog (OK msg:1)")
                n282 = call <vilib>:"General Error Handler.vi"("[error code] (0)"=5011, "[error source] (\" \")"="NOx Charting" ("[error source] (\" \")"), "type of dialog (OK msg:1)"=w419, "error in (no error)"=w423) -> ("error out"=w422:errorcluster)  [unwired: 7 in, 4 out]
              }
            }
            n283 = case shown="Error" w377 {
              selector: w377 -> [w412 w417]
              tunnel: [w412 w416] -> w369
              frame No Error {
              }
              frame Error {
                w413 = T8 0 items=["no dialog", "OK message", "continue or stop message", "OK message + warnings", "continue/stop + warnings"] ("type of dialog (OK msg:1)")
                n284 = call <vilib>:"General Error Handler.vi"("[error code] (0)"=5011, "[error source] (\" \")"="SO2 Charting" ("[error source] (\" \")"), "type of dialog (OK msg:1)"=w413, "error in (no error)"=w417) -> ("error out"=w416:errorcluster)  [unwired: 7 in, 4 out]
              }
            }
            n285 = case shown="Error" w376 {
              selector: w376 -> [w406 w411]
              tunnel: [w406 w410] -> w375
              frame No Error {
              }
              frame Error {
                w407 = T8 0 items=["no dialog", "OK message", "continue or stop message", "OK message + warnings", "continue/stop + warnings"] ("type of dialog (OK msg:1)")
                n286 = call <vilib>:"General Error Handler.vi"("[error code] (0)"=5011, "[error source] (\" \")"="O3 Charting" ("[error source] (\" \")"), "type of dialog (OK msg:1)"=w407, "error in (no error)"=w411) -> ("error out"=w410:errorcluster)  [unwired: 7 in, 4 out]
              }
            }
            n287 = Build Array (concatenate)(w368, w367, w364) -> (w363:dbl[])
            n288 = Merge Errors(w379, w369, w375) -> (w381:errorcluster)
            n289 = Get Date/Time In Seconds() -> (seconds since 1Jan1904=w361:timestamp)
            n290 = property on="Log Thermo Data?" class="Bool (strict)"() -> ("Value"=w359:bool)  [unwired: 2 in, 2 out]
            n291 = Format Date/Time String(seconds (now)=w361, UTC format=FALSE ("to UTC (F)")) -> (date/time string=w357:string)  [unwired: 1 in]
            n292 = Format Date/Time String(seconds (now)=w361, UTC format=TRUE ("to UTC (F)")) -> (date/time string=w356:string)  [unwired: 1 in]
            n293 = case shown="True" w359 {
              tunnel: w363 -> [_ w396]
              tunnel: w358 -> [w387 w391]
              tunnel: w357 -> [_ w390]
              tunnel: w356 -> [_ w389]
              tunnel: [w387 w388] -> _
              frame False {
              }
              frame True {
                n294 = Array Size(array=w396) -> (size(s)=w397:i32)
                n295 = for {
                  N: w397 -> [_]
                  shift-right: [w404] -> w395
                  shift-left: string[] [] -> [w402]
                  tunnel: w396 -> [w399] mode=indexing
                  i -> [w405]
                  n296 = Format Value(string ("")="", format string="%.3f", value (0)=w399) -> (output string=w403:string)
                  n297 = Insert Into Array(array=w402, index=w405, new element=w403) -> (w404:string[])
                }
                n298 = local read "Delimeter"() -> (w392:string)
                n299 = Build Array (concatenate)(w390, w389, w395) -> (w394:string[])
                n300 = call-poly <vilib>:"Write To Spreadsheet File.vi"("delimiter (\\t)"=w392, "append to file? (new file:F)"=TRUE, "1D data"=w394, "file path (dialog if empty)"=w391) -> ("new file path (Not A Path if cancelled)"=w388:path)  [unwired: 3 in, 1 out]
              }
            }
            n301 = property on="Stop Button" class="Bool (strict)"() -> ("Value"=w385:bool)  [unwired: 2 in, 2 out]
            n302 = Or(x=w381, y=w385) -> (x .or. y?=w386:bool)
          }
          n303 = Merge Errors(w298, w296, w261) -> (w297:errorcluster)
        }
        frame Error {
        }
      }
      n304 = call <vilib>:"DAQmx Clear Task.vi"("task in"=w119, "error in"=w120) -> ("error out"=w141:errorcluster)  [unwired: 13 in]
      n305 = call <vilib>:"DAQmx Clear Task.vi"("task in"=w168, "error in"=w141) -> ("error out"=w198:errorcluster)  [unwired: 13 in]
    }
    frame Error {
    }
  }
  n306 = call <vilib>:"General Error Handler.vi"("[user-defined codes]"=i32[] [5003, 5004, 5005, 5006, 5007, 5008, 5009, 5010, 5011], "[user-defined descriptions]"=string[] ["There is an error with the DAQ configuration. Check to make sure there are an equal number of Labels, Channels, and Boolean ON/OFF switches set.", "There is an error with the labels for either a MFC, RHT Probe, or TC. One or more of the instruments does not have an appropriate label. Please check them and try again.", "There is an error with one of the setup SubVI's. Please check to make sure everything is okidokie.", "There is an error with the Display Values SubVI. You may as well give up, because this thing is ugly. It's probably going to take three days to fix...", "There is an error with the MFC Sequence file. It is most likely an invalid Flow rate. The most likely error is either a flow rate out of range or a poorly chosen scale.", "There is an error with the PID Program. Check to make sure everything is set up correctly in the Sub VI.", "", "There is an error in the Thermo Gas Conc Read (SubVI).vi. Please check to make sure everything is configured correctly.", "There is an error with the charting of the Thermoscientific gas analyzers. Please check to make sure everything is configured correctly."], "error in (no error)"=w89) -> ("error out"=→"Error Out":errorcluster)  [unwired: 8 in, 4 out]
  "Scale for N2 MFC 2" <- "Scale for N2 MFC"
  "N2 MFC 2" <- "N2 MFC"
  "Scale for O2 MFC 2" <- "Scale for O2 MFC"
  "O2 MFC 2" <- "O2 MFC"
  "Scale for NOx MFC 2" <- "Scale for NOx MFC"
  "NOx MFC 2" <- "NOx MFC"
  "Scale for VOC MFC 2" <- "Scale for VOC MFC"
  "VOC MFC 2" <- "VOC MFC"
